vi "Pulse Read Delay.vi"(8 "error in (no error)":errorcluster, 11 "3300 in":refnum<class "3300.lvclass">) -> (0 "error out":errorcluster, 3 "3300 out":refnum<class "3300.lvclass">)   [LabVIEW 2019, in "3300.lvlib" / "3300.lvclass"]
uses:
  Library/3300.lvclass
  C:/Users/Public/Documents/Development/builds/Instruments/Electronic Load.lvlibp/Library/Electronic Load.lvclass
  builds/Instruments/Electronic Load.lvlibp/Accessors/Trigger/Read All Pulse.vi
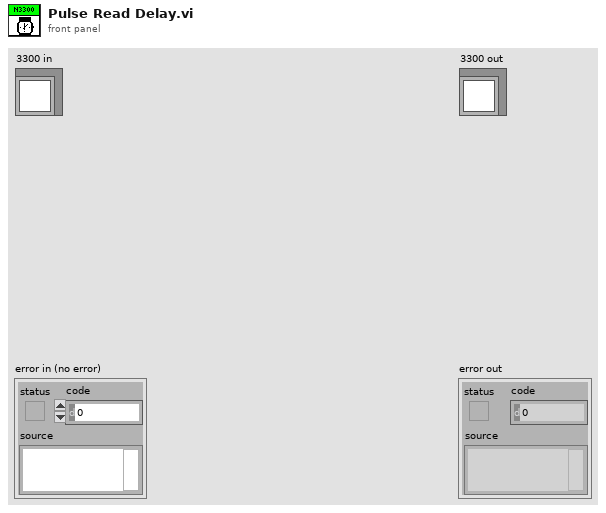
[diagram p1: front panel]
types:
  T1 = typedef "Electronic Load.lvlibp/Electronic Load.lvclass/Trigger Settings.ctl" = cluster{"Mode":T2, "Initial":dbl, "Transient":dbl, "Interval":dbl, "Width":dbl, "Delay":dbl, "Data Pts":i32, "Slew Rate":dbl}
  T2 = typedef "Electronic Load.lvlibp/Electronic Load.lvclass/E-Load Mode.ctl" = enum16{"Current", "Resistance", "Voltage"}
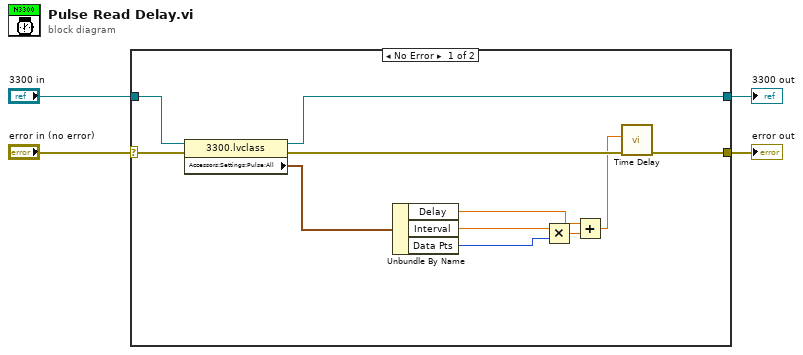
[diagram p0: block diagram]
diagram:
  n1 = case shown="No Error" "error in (no error)" {
    selector: "error in (no error)" -> [w9 w17]
    tunnel: [w7 w17] -> w3
    tunnel: [w10 w16] -> w1
    tunnel: "3300 in" -> [w15 w16]
    frame No Error {
      n2 = property class="3300.lvclass"(reference=w15, error in=w9) -> (reference out=w10:refnum<class "3300.lvclass">, error out=w8:errorcluster, "Accessors:Settings:Pulse:All"=w14:T1)
      n3 = Unbundle By Name(w14) -> ("Delay"=w5:dbl, "Interval"=w12:dbl, "Data Pts"=w13:i32)
      n4 = Multiply(x=w12, y=w13) -> (x*y=w11:dbl)
      n5 = Add(x=w5, y=w11) -> (x+y=w6:dbl)
      n6 = call "Time Delay"("error in (no error)"=w8, "Delay Time (s)"=w6) -> ("error out"=w7:errorcluster)  [unwired: 9 in]
    }
    frame Error {
    }
  }
  "error out" <- w3
  "3300 out" <- w1
